vi "更新列表.vi"(10 "AllTypes[]":T1 caption="VI服务器类信息数组", 11 "列表框引用 i":refnum<vi>) -> (3 "列表框引用 o":refnum<vi>)   [LabVIEW 2017]
uses:
  <vilib>/_script/All Supported PropertiesOrMethods TypeDefs/ASC_ArrayOfUniqueIDStringParentIDStringName.ctl
  <vilib>/_script/All Supported PropertiesOrMethods TypeDefs/ASC_UniqueIDStringParentIDStringName.ctl
  <vilib>/Utility/miscctls.llb/LVRowAndColumnUnsignedTypeDef.ctl
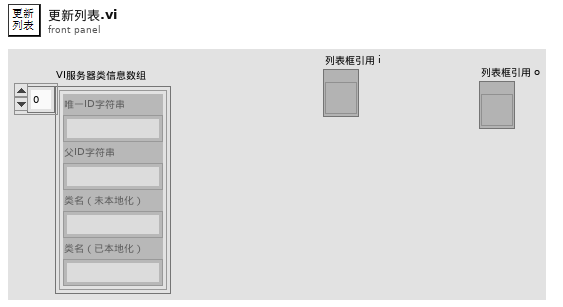
[diagram p1: front panel]
types:
  T1 = typedef "ASC_ArrayOfUniqueIDStringParentIDStringName.ctl" = T2[]
  T2 = typedef "ASC_UniqueIDStringParentIDStringName.ctl" = cluster{"Unique ID string":string, "Parent ID string":string, "Class Name (unlocalized)":string, "Class Name (localized)":string}
  T3 = typedef "LVRowAndColumnUnsignedTypeDef.ctl" = cluster{"Row":u32, "Column":u32}
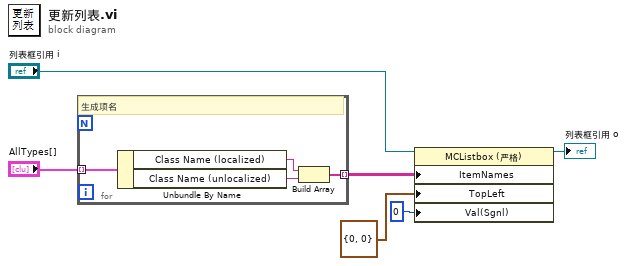
[diagram p0: block diagram]
diagram:
  n1 = for {
    tunnel: "AllTypes[]" -> [w10] mode=indexing
    tunnel: [w7] -> w1 mode=indexing
    # "生成项名"
    n2 = Unbundle By Name(w10) -> ("Class Name (localized)"=w9:string, "Class Name (unlocalized)"=w8:string)
    n3 = Build Array(w9, w8) -> (w7:string[])
  }
  n4 = property class="MCListbox (严格)"(reference="列表框引用 i", "ItemNames"=w1, "TopLeft"=T3 {"Row"=0, "Column"=0} ("左上可见单元格"), "Val(Sgnl)"=0 ("值(信号)")) -> (reference out=→"列表框引用 o":refnum<vi>)  [unwired: 1 in, 1 out]
